vi "Test_Make_data_frame_and_put_somewhere.vi"(6 "At least bits":u32=30, 8 "error in":errorcluster, 11 "VISA resource name in":refnum<visa-resource-name>) -> (0 "error out":errorcluster, 1 "High-speed channel":T1, 2 "Timestamp":timestamp, 3 "VISA resource name out":refnum<visa-resource-name>, 4 "Time to process, us":dbl format="%0.2f")   [LabVIEW 2018]
uses:
  <extravilib>/ChannelInstances/High Speed Stream-c(a[.](u16),stamp,str)/)Channel.ctl
  <vilib>/Analysis/baseanly.llb/Mean (DBL).vi
  <extravilib>/ChannelInstances/High Speed Stream-c(a[.](u16),stamp,str)/)Channel.vi
  Common_Resources.lvlib
  <vilib>/Analysis/NI_AALBase.lvlib
  <extravilib>/ChannelInstances/High Speed Stream-c(a[.](u16),stamp,str).lvlib
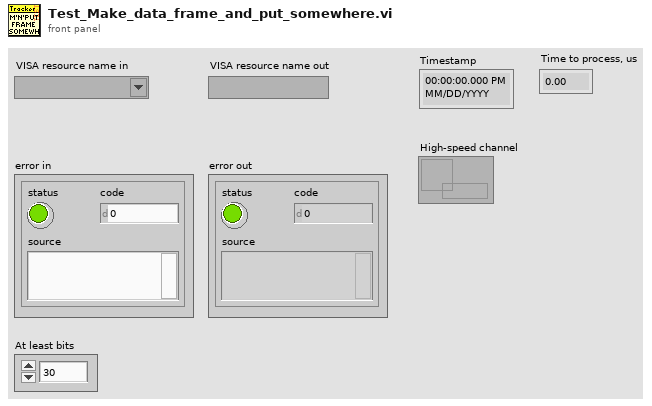
[diagram p1: front panel]
types:
  T1 = typedef "High Speed Stream-c(a[.](u16),stamp,str).lvlib/)Channel.ctl" = refnum<queue>
  T2 = cluster{u16[], "seconds since 1Jan1904":timestamp, "read buffer":string}
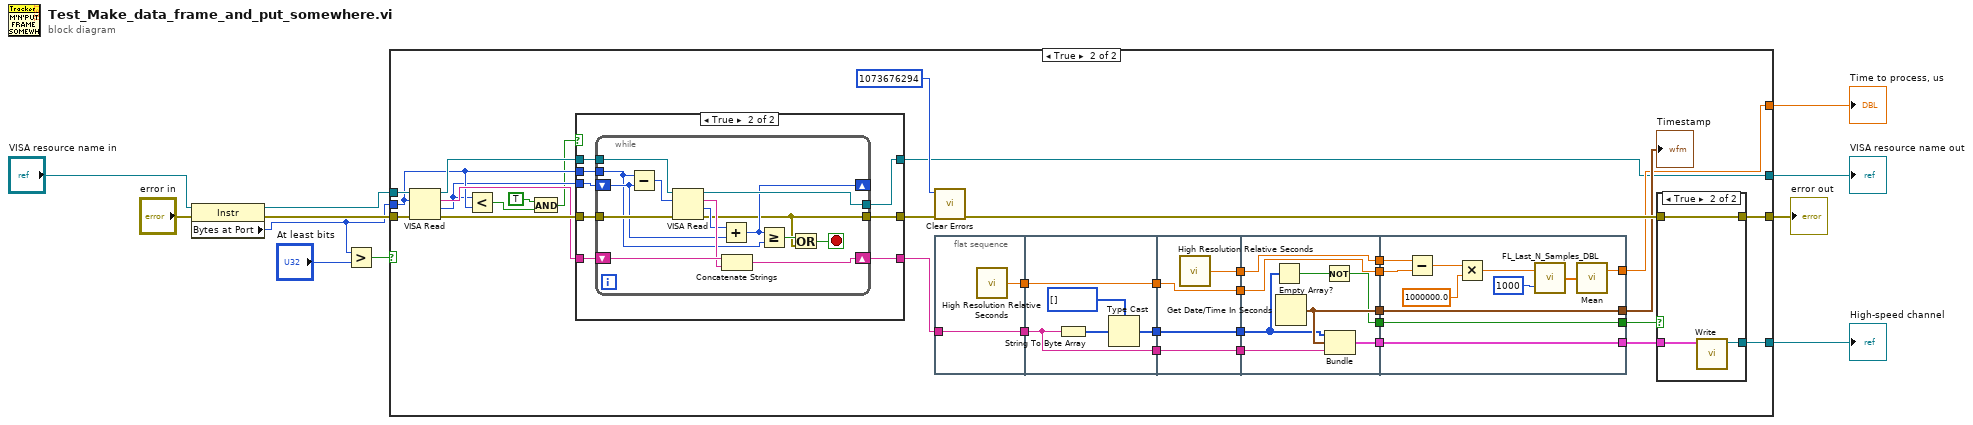
[diagram p0: block diagram]
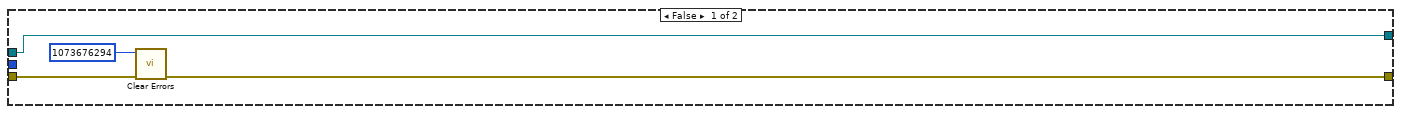
[diagram p2: hidden frame]
diagram:
  n1 = property class="Instr"(reference="VISA resource name in", error in="error in") -> (reference out=w8:refnum<visa-resource-name>, error out=w9:errorcluster, "Bytes at Port"=w4:u32)
  n2 = Greater?(x=w4, y="At least bits") -> (0:w3:bool)
  n3 = case shown="True" w3 {
    tunnel: [w13 w37] -> w11
    tunnel: [w12 w24] -> w10
    tunnel: w9 -> [w14 w32]
    tunnel: w8 -> [w12 w31]
    tunnel: [_ w30] -> w5
    tunnel: w4 -> [_ w19]
    tunnel: [_ w29] -> w1
    frame False {
      n4 = call <vilib>:"Clear Errors.vi"("error in (no error)"=w14, "specific error code to clear (0: all)"=1073676294) -> ("error out"=w13:errorcluster)  [unwired: 4 in, 1 out]
    }
    frame True {
      n5 = VISA Read(VISA resource name=w31, byte count=w19, error in (no error)=w32) -> (VISA resource name out=w25:refnum<visa-resource-name>, read buffer=w20:string, return count=w18:u32, error out=w22:errorcluster)
      n6 = Less?(x=w18, y=w19) -> (x < y?=w26:bool)
      n7 = And(x=TRUE, y=w26) -> (x .and. y?=w17:bool)
      n8 = case shown="True" w17 {
        tunnel: w25 -> [w53 w61]
        tunnel: [w53 w60] -> w24
        tunnel: [w52 w56] -> w23
        tunnel: w22 -> [w52 w59]
        tunnel: [w51 w57] -> w21
        tunnel: w20 -> [w51 w58]
        tunnel: w19 -> [_ w55]
        tunnel: w18 -> [_ w54]
        frame False {
        }
        frame True {
          n9 = while {
            tunnel: w61 -> [w75]
            tunnel: [w74] -> w60
            tunnel: w59 -> [w73]
            tunnel: [w62] -> w56
            shift-right: [w69] -> w57
            shift-left: w58 -> [w71]
            tunnel: w55 -> [w66]
            shift-right: [w64] -> _
            shift-left: w54 -> [w67]
            stop <- w63 stop-if-true
            n10 = Subtract(x=w66, y=w67) -> (x-y=w72:u32)
            n11 = VISA Read(VISA resource name=w75, byte count=w72, error in (no error)=w73) -> (VISA resource name out=w74:refnum<visa-resource-name>, read buffer=w70:string, return count=w68:u32, error out=w62:errorcluster)
            n12 = Add(x=w68, y=w67) -> (x+y=w64:u32)
            n13 = Concatenate Strings(w71, w70) -> (w69:string)
            n14 = Greater Or Equal?(x=w64, y=w66) -> (x >= y?=w65:bool)
            n15 = Or(x=w65, y=w62) -> (x .or. y?=w63:bool)
          }
        }
      }
      n16 = call <vilib>:"Clear Errors.vi"("error in (no error)"=w23, "specific error code to clear (0: all)"=1073676294) -> ("error out"=w36:errorcluster)  [unwired: 4 in, 1 out]
      n17 = flat-sequence {
        tunnel: w21 -> [w77]
        tunnel: [w77] -> w50
        tunnel: [w76] -> w49
        tunnel: w50 -> [w78]
        tunnel: [w79] -> w48
        tunnel: w49 -> [w82]
        tunnel: [w82] -> w47
        tunnel: [w78] -> w28
        tunnel: w48 -> [w86]
        tunnel: [w86] -> w46
        tunnel: w47 -> [w85]
        tunnel: [w85] -> w45
        tunnel: [w84] -> w44
        tunnel: w28 -> [w83]
        tunnel: [w83] -> w27
        tunnel: w46 -> [w90]
        tunnel: w45 -> [w94]
        tunnel: [w88] -> w43
        tunnel: [w92] -> w42
        tunnel: [w91] -> w41
        tunnel: [w94] -> w40
        tunnel: [w93] -> w39
        tunnel: w44 -> [w93]
        tunnel: w27 -> [w87]
        tunnel: [w95] -> w30
        tunnel: [w103] -> w34
        tunnel: [w104] -> w35
        tunnel: [w105] -> w38
        tunnel: w43 -> [w105]
        tunnel: w42 -> [w104]
        tunnel: w41 -> [w103]
        tunnel: w40 -> [w97]
        tunnel: w39 -> [w96]
        frame #0 {
          n18 = call <vilib>:"High Resolution Relative Seconds.vi"() -> ("relative seconds"=w76:dbl)
        }
        frame #1 {
          n19 = String To Byte Array(string=w78) -> (unsigned byte array=w81:u8[])
          n20 = Type Cast(type=u16[] [], x=w81) -> (*(type *) &x=w79:u16[])
        }
        frame #2 {
          n21 = call <vilib>:"High Resolution Relative Seconds.vi"() -> ("relative seconds"=w84:dbl)
        }
        frame #3 {
          n22 = Empty Array?(array=w90) -> (empty?=w89:bool)
          n23 = Get Date/Time In Seconds ("Current time")() -> (seconds since 1Jan1904=w91:timestamp)
          n24 = Not(x=w89) -> (.not. x?=w88:bool)
          n25 = Bundle(w90, "seconds since 1Jan1904"=w91, "read buffer"=w87) -> (w92:T2)  [unwired: 1 in]
        }
        frame #4 {
          n26 = Subtract(x=w96, y=w97) -> (x-y=w100:dbl)
          n27 = Multiply(x=w100, y=1000000.0) -> (x*y=w101:dbl)
          n28 = call "FL_Last_N_Samples_DBL.vi"("BufferLengthSamples"=1000, "Input sample"=w101) -> ("Output Array"=w102:dbl[])
          n29 = call-poly <vilib>:"Mean.vi"("X"=w102) -> ("mean"=w95:dbl)  [unwired: 1 out]
        }
      }
      n30 = case shown="True" w38 {
        tunnel: w35 -> [_ w108]
        tunnel: w36 -> [w106 w109]
        tunnel: [w106 w109] -> w37
        tunnel: [_ w107] -> w29
        frame False {
        }
        frame True {
          n31 = call <extravilib>:"Write.vi"("element"=w108) -> ("channel"=w107:T1)  [unwired: 8 in, 2 out]
        }
      }
      "Timestamp" <- w34
    }
  }
  "error out" <- w11
  "VISA resource name out" <- w10
  "Time to process, us" <- w5
  "High-speed channel" <- w1
